vi "Movefortime.vi"(8 "error in (no error)":errorcluster) -> (0 "error out":errorcluster)   [LabVIEW 2017]
panel:
  in  "Setpoint":dbl
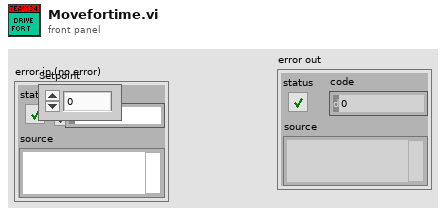
[diagram p1: front panel]
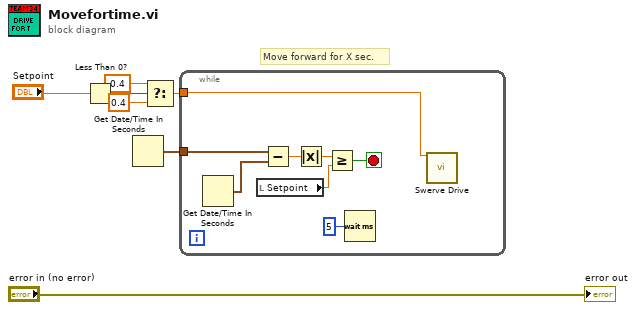
[diagram p0: block diagram]
diagram:
  # "Move forward for X sec."
  n1 = Less Than 0?(x="Setpoint") -> (x < 0?=w5:bool)
  n2 = Get Date/Time In Seconds() -> (seconds since 1Jan1904=w7:timestamp)
  n3 = Select(t=-0.4, s=w5, f=0.4) -> (s? t:f=w2:dbl)
  n4 = while {
    tunnel: w7 -> [w15]
    tunnel: w2 -> [w8]
    stop <- w10 stop-if-true
    n5 = Get Date/Time In Seconds() -> (seconds since 1Jan1904=w14:timestamp)
    n6 = local read "Setpoint"() -> (w11:dbl)
    n7 = Subtract(x=w15, y=w14) -> (x-y=w13:dbl)
    n8 = Absolute Value(x=w13) -> (abs(x)=w12:dbl)
    n9 = Greater Or Equal?(x=w12, y=w11) -> (x >= y?=w10:bool)
    n10 = Wait (ms)(milliseconds to wait=u32 5) -> ()  [unwired: 1 out]
    n11 = call "Swerve Drive.vi"("X"=w8) -> ()  [unwired: 10 in, 5 out]
  }
  "error out" <- "error in (no error)"
